vi "2100_Sequenced_Load Line w_Telegram Writes.vi"(0 "Semiconductor Module Context":T2, 1 "Published_Data_ID":string="HV_", 2 "Reg0_State":string="State00", 3 "HV_Load_Steps_uA":dbl[](array[numeric])=[0.0, 2.0, 4.0, 6.0, 8.0, 10.0, 12.0, 14.0, 16.0, 18.0, 20.0] format="%#_6p", 4 "USID":T1 max=15, 6 "Measurement:Aperture Time":dbl=2.5e-05 format="%#_13p", 8 "current level range":dbl=0.0001 format="%#_13p") -> ()   [LabVIEW 2013]
uses:
  <vilib>/NI_TestStand_SemiconductorModule/NI_TestStand_Semiconductor_Module.lvlibp/PinMap/General/SemiconductorModuleContext.ctl
  Controls/USID.ctl
  <instrlib>/niHSDIO/niHSDIO.llb/niHSDIO_ctl Generation Mode Values (Ring).ctl
  <instrlib>/niDCPower/nidcpower.llb/niDCPower Source Mode.ctl
  <instrlib>/niDCPower/nidcpower.llb/niDCPower Output Function.ctl
  <instrlib>/niDCPower/nidcpower.llb/niDCPower Sense.ctl
  <instrlib>/niDCPower/nidcpower.llb/niDCPower Wait For Event - Event.ctl
  <instrlib>/niHSDIO/niHSDIO.llb/niHSDIO_ctl Trigger SW - TrigName Values (Ring).ctl
  <instrlib>/niHSDIO/niHSDIO.llb/niHSDIO_ctl Trigger SW - TrigIdentifier Values (Ring).ctl
  <vilib>/NI_TestStand_SemiconductorModule/NI_TestStand_Semiconductor_Module.lvlibp/PinMap/HSDIO/PinsToNIHSDIOSessions.vi
  <vilib>/NI_TestStand_SemiconductorModule/NI_TestStand_Semiconductor_Module.lvlibp/PinMap/DC Power/PinsToNIDCPowerSessions.vi
  <vilib>/NI_TestStand_SemiconductorModule/NI_TestStand_Semiconductor_Module.lvlibp/PinMap/Deprecated/PublishDataDoubleMultiplePinsSingleInstrument.vi
  <vilib>/NI_TestStand_SemiconductorModule/NI_TestStand_Semiconductor_Module.lvlibp
panel:
  in  "Source:Transient Response":i32(ring)=1039 items=["Slow"=1041, "Normal"=1038, "Fast"=1039, "Custom"=1042]
  out "actual count":i32
  out "Avg_Meas_HV":dbl[](array[numeric])
  in  "Scratch Pad":string="Script test\nrepeat 10\nGenerate BRGu2rAd133\nend repeat\nend Script"
  in  "Num_Iterations_Per_Load_Step":i32=20
  in  "Script_Run":string="Script LoadLine\nRepeat Until ScriptTrigger0\nGenerate BRGu2rAd133\nend repeat\nend Script"
  in  "HSDIO_Pins":string[](array[string])=["CLK", "SDA"]
  out "HV Load Current":cluster{"X":dbl, "Y":dbl}[](graph)=[{"X"=0.0, "Y"=-1.7168055552671937e-06}, {"X"=2.4999999999999998e-05, "Y"=2.162222413914116e-07}, {"X"=4.9999999999999996e-05, "Y"=1.90283128600777e-07}, {"X"=7.5e-05, "Y"=1.7674967844914135e-07}, {"X"=9.999999999999999e-05, "Y"=1.7674967844914135e-07}, {"X"=0.000125, "Y"=-9.183319963206986e-07}, {"X"=0.00015, "Y"=1.993054287018673e-07}, {"X"=0.00017499999999999997, "Y"=1.891553410881407e-07}, {"X"=0.00019999999999999998, "Y"=1.7900525347441391e-07}, {"X"=0.000225, "Y"=-1.190128786866045e-06}, {"X"=0.00025, "Y"=2.2298896646722935e-07}, {"X"=0.00027499999999999996, "Y"=1.993054287018673e-07}, {"X"=0.0003, "Y"=1.812608284996865e-07}, {"X"=0.000325, "Y"=1.812608284996865e-07}, {"X"=0.00034999999999999994, "Y"=-9.093096962196083e-07}, {"X"=0.00037499999999999995, "Y"=1.891553410881407e-07}, {"X"=0.00039999999999999996, "Y"=1.8689976606286793e-07}, {"X"=0.000425, "Y"=1.880275535755044e-07}, {"X"=0.00045, "Y"=-1.5837266287761109e-06}, {"X"=0.00047499999999999994, "Y"=2.3426684159359224e-07}, {"X"=0.0005, "Y"=1.8013304098705022e-07}, {"X"=0.000525, "Y"=1.7900525347441391e-07}, {"X"=0.0005499999999999999, "Y"=1.8351640352495906e-07}, {"X"=0.000575, "Y"=-6.634520184648964e-07}, {"X"=0.0006, "Y"=2.1283887885350274e-07}, {"X"=0.0006249999999999999, "Y"=1.9141091611341327e-07}, {"X"=0.00065, "Y"=1.7449410342386876e-07}, {"X"=0.0006749999999999999, "Y"=-9.792325220030581e-07}, {"X"=0.0006999999999999999, "Y"=1.812608284996865e-07}, {"X"=0.000725, "Y"=1.7562189093650507e-07}, {"X"=0.0007499999999999999, "Y"=1.7787746596177763e-07}, {"X"=0.000775, "Y"=1.8013304098705022e-07}, {"X"=0.0007999999999999999, "Y"=6.763595465470189e-07}, {"X"=0.0008249999999999999, "Y"=2.094555163155939e-07}, {"X"=0.00085, "Y"=1.993054287018673e-07}, {"X"=0.0008749999999999999, "Y"=1.8689976606286793e-07}, {"X"=0.0009, "Y"=-9.453988966239696e-07}, {"X"=0.0009249999999999999, "Y"=1.9141091611341327e-07}, {"X"=0.0009499999999999999, "Y"=1.8013304098705022e-07}, {"X"=0.000975, "Y"=1.711107408859599e-07}, {"X"=0.001, "Y"=-3.0707116447182816e-07}, {"X"=0.0010249999999999999, "Y"=1.5419392819641557e-07}, {"X"=0.00105, "Y"=1.8238861601232278e-07}, {"X"=0.001075, "Y"=1.711107408859599e-07}, {"X"=0.0010999999999999998, "Y"=1.6772737834805105e-07}, {"X"=0.001125, "Y"=-9.386321715481518e-07}, {"X"=0.00115, "Y"=1.8351640352495906e-07}, {"X"=0.0011749999999999998, "Y"=1.8238861601232278e-07}, {"X"=0.0012, "Y"=1.8464419103759537e-07}, {"X"=0.001225, "Y"=-1.4810979651262086e-06}, {"X"=0.0012499999999999998, "Y"=-1.13875834761234e-05}, {"X"=0.0012749999999999999, "Y"=-1.2762356454027042e-05}, {"X"=0.0013, "Y"=-1.1686447166972018e-05}, {"X"=0.0013249999999999998, "Y"=-1.2103728546647446e-05}, {"X"=0.0013499999999999999, "Y"=-1.1891704494271823e-05}, {"X"=0.001375, "Y"=-1.2064255983705175e-05}, {"X"=0.0013999999999999998, "Y"=-1.2136434384513899e-05}, {"X"=0.0014249999999999998, "Y"=-1.1844337418741099e-05}, {"X"=0.00145, "Y"=-1.1872532106557007e-05}, {"X"=0.001475, "Y"=-1.2131923234463352e-05}, {"X"=0.0014999999999999998, "Y"=-1.2065383771217813e-05}, {"X"=0.0015249999999999999, "Y"=-1.181050379336201e-05}, {"X"=0.00155, "Y"=-1.1981927495282728e-05}, {"X"=0.0015749999999999998, "Y"=-1.2099217396596903e-05}, {"X"=0.0015999999999999999, "Y"=-1.2056361471116722e-05}, {"X"=0.001625, "Y"=-1.2046211383502995e-05}, {"X"=0.0016499999999999998, "Y"=-1.1473295327083758e-05}, {"X"=0.0016749999999999998, "Y"=-1.2156734559741353e-05}, {"X"=0.0017, "Y"=-1.2094706246546357e-05}, {"X"=0.0017249999999999998, "Y"=-1.2060872621167267e-05}, {"X"=0.0017499999999999998, "Y"=-1.2048466958528269e-05}, {"X"=0.0017749999999999999, "Y"=-1.165825247915611e-05}, {"X"=0.0018, "Y"=-1.2139817747051807e-05}, {"X"=0.0018249999999999998, "Y"=-1.2071022708780994e-05}, {"X"=0.0018499999999999999, "Y"=-1.1707875129712107e-05}, {"X"=0.001875, "Y"=-1.2161245709791896e-05}, {"X"=0.0018999999999999998, "Y"=-1.2092450671521083e-05}, {"X"=0.0019249999999999998, "Y"=-1.2056361471116722e-05}, {"X"=0.00195, "Y"=-1.205410589609145e-05}, {"X"=0.0019749999999999998, "Y"=-1.1493595502311211e-05}, {"X"=0.002, "Y"=-1.2143201109589716e-05}, {"X"=0.002025, "Y"=-1.2102600759134812e-05}, {"X"=0.0020499999999999997, "Y"=-1.2065383771217813e-05}, {"X"=0.002075, "Y"=-1.192328254462564e-05}, {"X"=0.0021, "Y"=-1.1752986630217559e-05}, {"X"=0.0021249999999999997, "Y"=-1.212741208441281e-05}, {"X"=0.00215, "Y"=-1.2063128196192539e-05}, {"X"=0.002175, "Y"=-1.2048466958528269e-05}, {"X"=0.0021999999999999997, "Y"=-1.2043955808477724e-05}, {"X"=0.002225, "Y"=-1.1619907703726478e-05}, {"X"=0.00225, "Y"=-1.219056818512044e-05}, {"X"=0.0022749999999999997, "Y"=-1.2086811733957902e-05}, {"X"=0.0023, "Y"=-1.2062000408679905e-05}, {"X"=0.002325, "Y"=-1.205410589609145e-05}, {"X"=0.0023499999999999997, "Y"=-1.1803737068286193e-05}, {"X"=0.002375, "Y"=-1.2008994395585998e-05}, {"X"=0.0024, "Y"=-1.2109367484210629e-05}, {"X"=0.0024249999999999996, "Y"=-1.2065383771217813e-05}, {"X"=0.00245, "Y"=-1.2043955808477724e-05}, {"X"=0.0024749999999999998, "Y"=-1.1533068065253484e-05}, {"X"=0.0024999999999999996, "Y"=-1.2196207122683623e-05}, {"X"=0.002525, "Y"=-1.2089067308983174e-05}, {"X"=0.0025499999999999997, "Y"=-1.2064255983705175e-05}, {"X"=0.0025749999999999996, "Y"=-1.2047339171015633e-05}, {"X"=0.0026, "Y"=-1.1910876881986638e-05}, {"X"=0.0026249999999999997, "Y"=-1.1693213892047838e-05}, {"X"=0.0026499999999999996, "Y"=-1.2147712259640262e-05}, {"X"=0.002675, "Y"=-1.2067639346243084e-05}, {"X"=0.0026999999999999997, "Y"=-1.2051850321066179e-05}, {"X"=0.0027249999999999996, "Y"=-1.184772078127901e-05}, {"X"=0.00275, "Y"=-1.1878171044120186e-05}, {"X"=0.0027749999999999997, "Y"=-1.2128539871925444e-05}, {"X"=0.0027999999999999995, "Y"=-1.206989492126836e-05}, {"X"=0.002825, "Y"=-1.2056361471116722e-05}, {"X"=0.0028499999999999997, "Y"=-1.1917643607062459e-05}, {"X"=0.002875, "Y"=-1.1721408579863744e-05}, {"X"=0.0029, "Y"=-1.2137562172026535e-05}, {"X"=0.0029249999999999996, "Y"=-1.2063128196192539e-05}, {"X"=0.00295, "Y"=-1.2047339171015633e-05}, {"X"=0.0029749999999999998, "Y"=-1.1780053530520832e-05}, {"X"=0.0029999999999999996, "Y"=-1.1910876881986638e-05}, {"X"=0.003025, "Y"=-1.2121773146849627e-05}, {"X"=0.0030499999999999998, "Y"=-1.2063128196192539e-05}, {"X"=0.0030749999999999996, "Y"=-1.2042828020965086e-05}, {"X"=0.0031, "Y"=-1.2037189083401907e-05}, {"X"=0.0031249999999999997, "Y"=-1.1581562928296841e-05}, {"X"=0.0031499999999999996, "Y"=-1.2186057035069897e-05}, {"X"=0.003175, "Y"=-1.2082300583907356e-05}, {"X"=0.0031999999999999997, "Y"=-1.2049594746040903e-05}, {"X"=0.0032249999999999996, "Y"=-1.2046211383502995e-05}, {"X"=0.00325, "Y"=-1.1610885403625385e-05}, {"X"=0.0032749999999999997, "Y"=-1.2252596498315437e-05}, {"X"=0.0032999999999999995, "Y"=-1.2089067308983174e-05}, {"X"=0.003325, "Y"=-1.2067639346243084e-05}, {"X"=0.0033499999999999997, "Y"=-1.1626674428802295e-05}, {"X"=0.0033749999999999995, "Y"=-1.2208612785322621e-05}, {"X"=0.0034, "Y"=-1.2101472971622174e-05}, {"X"=0.0034249999999999997, "Y"=-1.2078917221369447e-05}, {"X"=0.0034499999999999995, "Y"=-1.1853359718842188e-05}, {"X"=0.003475, "Y"=-1.2004483245535455e-05}, {"X"=0.0034999999999999996, "Y"=-1.213305102197599e-05}, {"X"=0.0035249999999999995, "Y"=-1.2089067308983174e-05}, {"X"=0.0035499999999999998, "Y"=-1.2080045008882085e-05}, {"X"=0.0035749999999999996, "Y"=-1.1715769642300562e-05}, {"X"=0.0036, "Y"=-1.2038316870914541e-05}, {"X"=0.0036249999999999998, "Y"=-1.2115006421773808e-05}, {"X"=0.0036499999999999996, "Y"=-1.2073278283806268e-05}, {"X"=0.003675, "Y"=-1.2049594746040903e-05}]
  out "current measurements":dbl[](array[numeric])=[-1.7168055552671937e-06, 2.162222413914116e-07, 1.90283128600777e-07, 1.7674967844914135e-07, 1.7674967844914135e-07, -9.183319963206986e-07, 1.993054287018673e-07, 1.891553410881407e-07, 1.7900525347441391e-07, -1.190128786866045e-06, 2.2298896646722935e-07, 1.993054287018673e-07, 1.812608284996865e-07, 1.812608284996865e-07, -9.093096962196083e-07, 1.891553410881407e-07, 1.8689976606286793e-07, 1.880275535755044e-07, -1.5837266287761109e-06, 2.3426684159359224e-07, 1.8013304098705022e-07, 1.7900525347441391e-07, 1.8351640352495906e-07, -6.634520184648964e-07, 2.1283887885350274e-07, 1.9141091611341327e-07, 1.7449410342386876e-07, -9.792325220030581e-07, 1.812608284996865e-07, 1.7562189093650507e-07, 1.7787746596177763e-07, 1.8013304098705022e-07, 6.763595465470189e-07, 2.094555163155939e-07, 1.993054287018673e-07, 1.8689976606286793e-07, -9.453988966239696e-07, 1.9141091611341327e-07, 1.8013304098705022e-07, 1.711107408859599e-07, -3.0707116447182816e-07, 1.5419392819641557e-07, 1.8238861601232278e-07, 1.711107408859599e-07, 1.6772737834805105e-07, -9.386321715481518e-07, 1.8351640352495906e-07, 1.8238861601232278e-07, 1.8464419103759537e-07, -1.4810979651262086e-06, -1.13875834761234e-05, -1.2762356454027042e-05, -1.1686447166972018e-05, -1.2103728546647446e-05, -1.1891704494271823e-05, -1.2064255983705175e-05, -1.2136434384513899e-05, -1.1844337418741099e-05, -1.1872532106557007e-05, -1.2131923234463352e-05, -1.2065383771217813e-05, -1.181050379336201e-05, -1.1981927495282728e-05, -1.2099217396596903e-05, -1.2056361471116722e-05, -1.2046211383502995e-05, -1.1473295327083758e-05, -1.2156734559741353e-05, -1.2094706246546357e-05, -1.2060872621167267e-05, -1.2048466958528269e-05, -1.165825247915611e-05, -1.2139817747051807e-05, -1.2071022708780994e-05, -1.1707875129712107e-05, -1.2161245709791896e-05, -1.2092450671521083e-05, -1.2056361471116722e-05, -1.205410589609145e-05, -1.1493595502311211e-05, -1.2143201109589716e-05, -1.2102600759134812e-05, -1.2065383771217813e-05, -1.192328254462564e-05, -1.1752986630217559e-05, -1.212741208441281e-05, -1.2063128196192539e-05, -1.2048466958528269e-05, -1.2043955808477724e-05, -1.1619907703726478e-05, -1.219056818512044e-05, -1.2086811733957902e-05, -1.2062000408679905e-05, -1.205410589609145e-05, -1.1803737068286193e-05, -1.2008994395585998e-05, -1.2109367484210629e-05, -1.2065383771217813e-05, -1.2043955808477724e-05, -1.1533068065253484e-05, -1.2196207122683623e-05, -1.2089067308983174e-05, -1.2064255983705175e-05, -1.2047339171015633e-05, -1.1910876881986638e-05, -1.1693213892047838e-05, -1.2147712259640262e-05, -1.2067639346243084e-05, -1.2051850321066179e-05, -1.184772078127901e-05, -1.1878171044120186e-05, -1.2128539871925444e-05, -1.206989492126836e-05, -1.2056361471116722e-05, -1.1917643607062459e-05, -1.1721408579863744e-05, -1.2137562172026535e-05, -1.2063128196192539e-05, -1.2047339171015633e-05, -1.1780053530520832e-05, -1.1910876881986638e-05, -1.2121773146849627e-05, -1.2063128196192539e-05, -1.2042828020965086e-05, -1.2037189083401907e-05, -1.1581562928296841e-05, -1.2186057035069897e-05, -1.2082300583907356e-05, -1.2049594746040903e-05, -1.2046211383502995e-05, -1.1610885403625385e-05, -1.2252596498315437e-05, -1.2089067308983174e-05, -1.2067639346243084e-05, -1.1626674428802295e-05, -1.2208612785322621e-05, -1.2101472971622174e-05, -1.2078917221369447e-05, -1.1853359718842188e-05, -1.2004483245535455e-05, -1.213305102197599e-05, -1.2089067308983174e-05, -1.2080045008882085e-05, -1.1715769642300562e-05, -1.2038316870914541e-05, -1.2115006421773808e-05, -1.2073278283806268e-05, -1.2049594746040903e-05, -1.159509637844848e-05] format="%#_6p"
  out "voltage measurements":dbl[](array[numeric])=[41.400019787154584, 41.491719884993515, 41.449526588441856, 41.407333291890204, 41.36626514991326, 41.397206900717805, 41.46246586605103, 41.421960301361445, 41.38032958209715, 41.350512985867304, 41.48159349382112, 41.4377124654074, 41.39383143699368, 41.35220071772937, 41.448401433867154, 41.45065174301657, 41.40902102375227, 41.365702572625906, 41.349387831292596, 41.47034194807401, 41.42814865152235, 41.384267623108634, 41.34151174926962, 41.47259225722343, 41.44052535184417, 41.39889463257987, 41.35276329501673, 41.397206900717805, 41.458527825039546, 41.417459683062596, 41.37189092278681, 41.33082278080987, 41.47990576195905, 41.43714988812004, 41.394394014281026, 41.35220071772937, 41.391581127844255, 41.45627751589013, 41.41127133290169, 41.369640613637394, 41.33194793538458, 41.47202967993607, 41.429273806097065, 41.38764308683277, 41.34657494485582, 41.47371741179815, 41.44727627929244, 41.40508298274078, 41.36457741805119, 41.350512985867304, 41.350512985867304, 41.17555144949977, 41.243060723982424, 41.27569020664904, 41.266126392763994, 41.25993804260308, 41.29931845271796, 41.317320925913336, 41.247561342281266, 41.273439897499614, 41.29650556628119, 41.30494422559152, 41.243060723982424, 41.27569020664904, 41.297068143568545, 41.31338288490185, 41.27906567037317, 41.238560105683575, 41.27456505207432, 41.29313010255706, 41.30944484389036, 41.25825031074102, 41.26556381547664, 41.29031721612028, 41.27794051579846, 41.243060723982424, 41.27625278393639, 41.29481783441912, 41.310007421177716, 41.289754638832925, 41.23124660094796, 41.26893927920077, 41.29144237069499, 41.30156876186739, 41.24249814669507, 41.257687733453665, 41.28412886595937, 41.298193298143254, 41.31338288490185, 41.26556381547664, 41.231809178235316, 41.26837670191342, 41.286941752396146, 41.30156876186739, 41.307194534740944, 41.24474845584449, 41.273439897499614, 41.297068143568545, 41.31113257575243, 41.28581659782144, 41.23912268297094, 41.27794051579846, 41.29594298899383, 41.30944484389036, 41.32069638963747, 41.25374969244218, 41.2610631971778, 41.288629484258216, 41.30494422559152, 41.31113257575243, 41.238560105683575, 41.26162577446515, 41.2875043296835, 41.3077571120283, 41.31450803947656, 41.24924907414333, 41.262188351752506, 41.289754638832925, 41.30606938016623, 41.310007421177716, 41.227308559936475, 41.25825031074102, 41.28581659782144, 41.29875587543061, 41.31394546218921, 41.27456505207432, 41.24362330126978, 41.27681536122375, 41.298193298143254, 41.311695153039786, 41.27850309308581, 41.257687733453665, 41.2875043296835, 41.305506802878874, 41.27794051579846, 41.25712515616631, 41.28581659782144, 41.304381648304165, 41.30888226660301, 41.24418587855713, 41.274002474786975, 41.298193298143254, 41.31394546218921, 41.310007421177716, 41.238560105683575, 41.26950185648813, 41.29144237069499, 41.30831968931565, 41.285254020534076]
  out "HV Voltage":cluster{"X":dbl, "Y":dbl}[](graph)=[{"X"=0.0, "Y"=41.400019787154584}, {"X"=2.4999999999999998e-05, "Y"=41.491719884993515}, {"X"=4.9999999999999996e-05, "Y"=41.449526588441856}, {"X"=7.5e-05, "Y"=41.407333291890204}, {"X"=9.999999999999999e-05, "Y"=41.36626514991326}, {"X"=0.000125, "Y"=41.397206900717805}, {"X"=0.00015, "Y"=41.46246586605103}, {"X"=0.00017499999999999997, "Y"=41.421960301361445}, {"X"=0.00019999999999999998, "Y"=41.38032958209715}, {"X"=0.000225, "Y"=41.350512985867304}, {"X"=0.00025, "Y"=41.48159349382112}, {"X"=0.00027499999999999996, "Y"=41.4377124654074}, {"X"=0.0003, "Y"=41.39383143699368}, {"X"=0.000325, "Y"=41.35220071772937}, {"X"=0.00034999999999999994, "Y"=41.448401433867154}, {"X"=0.00037499999999999995, "Y"=41.45065174301657}, {"X"=0.00039999999999999996, "Y"=41.40902102375227}, {"X"=0.000425, "Y"=41.365702572625906}, {"X"=0.00045, "Y"=41.349387831292596}, {"X"=0.00047499999999999994, "Y"=41.47034194807401}, {"X"=0.0005, "Y"=41.42814865152235}, {"X"=0.000525, "Y"=41.384267623108634}, {"X"=0.0005499999999999999, "Y"=41.34151174926962}, {"X"=0.000575, "Y"=41.47259225722343}, {"X"=0.0006, "Y"=41.44052535184417}, {"X"=0.0006249999999999999, "Y"=41.39889463257987}, {"X"=0.00065, "Y"=41.35276329501673}, {"X"=0.0006749999999999999, "Y"=41.397206900717805}, {"X"=0.0006999999999999999, "Y"=41.458527825039546}, {"X"=0.000725, "Y"=41.417459683062596}, {"X"=0.0007499999999999999, "Y"=41.37189092278681}, {"X"=0.000775, "Y"=41.33082278080987}, {"X"=0.0007999999999999999, "Y"=41.47990576195905}, {"X"=0.0008249999999999999, "Y"=41.43714988812004}, {"X"=0.00085, "Y"=41.394394014281026}, {"X"=0.0008749999999999999, "Y"=41.35220071772937}, {"X"=0.0009, "Y"=41.391581127844255}, {"X"=0.0009249999999999999, "Y"=41.45627751589013}, {"X"=0.0009499999999999999, "Y"=41.41127133290169}, {"X"=0.000975, "Y"=41.369640613637394}, {"X"=0.001, "Y"=41.33194793538458}, {"X"=0.0010249999999999999, "Y"=41.47202967993607}, {"X"=0.00105, "Y"=41.429273806097065}, {"X"=0.001075, "Y"=41.38764308683277}, {"X"=0.0010999999999999998, "Y"=41.34657494485582}, {"X"=0.001125, "Y"=41.47371741179815}, {"X"=0.00115, "Y"=41.44727627929244}, {"X"=0.0011749999999999998, "Y"=41.40508298274078}, {"X"=0.0012, "Y"=41.36457741805119}, {"X"=0.001225, "Y"=41.350512985867304}, {"X"=0.0012499999999999998, "Y"=41.350512985867304}, {"X"=0.0012749999999999999, "Y"=41.17555144949977}, {"X"=0.0013, "Y"=41.243060723982424}, {"X"=0.0013249999999999998, "Y"=41.27569020664904}, {"X"=0.0013499999999999999, "Y"=41.266126392763994}, {"X"=0.001375, "Y"=41.25993804260308}, {"X"=0.0013999999999999998, "Y"=41.29931845271796}, {"X"=0.0014249999999999998, "Y"=41.317320925913336}, {"X"=0.00145, "Y"=41.247561342281266}, {"X"=0.001475, "Y"=41.273439897499614}, {"X"=0.0014999999999999998, "Y"=41.29650556628119}, {"X"=0.0015249999999999999, "Y"=41.30494422559152}, {"X"=0.00155, "Y"=41.243060723982424}, {"X"=0.0015749999999999998, "Y"=41.27569020664904}, {"X"=0.0015999999999999999, "Y"=41.297068143568545}, {"X"=0.001625, "Y"=41.31338288490185}, {"X"=0.0016499999999999998, "Y"=41.27906567037317}, {"X"=0.0016749999999999998, "Y"=41.238560105683575}, {"X"=0.0017, "Y"=41.27456505207432}, {"X"=0.0017249999999999998, "Y"=41.29313010255706}, {"X"=0.0017499999999999998, "Y"=41.30944484389036}, {"X"=0.0017749999999999999, "Y"=41.25825031074102}, {"X"=0.0018, "Y"=41.26556381547664}, {"X"=0.0018249999999999998, "Y"=41.29031721612028}, {"X"=0.0018499999999999999, "Y"=41.27794051579846}, {"X"=0.001875, "Y"=41.243060723982424}, {"X"=0.0018999999999999998, "Y"=41.27625278393639}, {"X"=0.0019249999999999998, "Y"=41.29481783441912}, {"X"=0.00195, "Y"=41.310007421177716}, {"X"=0.0019749999999999998, "Y"=41.289754638832925}, {"X"=0.002, "Y"=41.23124660094796}, {"X"=0.002025, "Y"=41.26893927920077}, {"X"=0.0020499999999999997, "Y"=41.29144237069499}, {"X"=0.002075, "Y"=41.30156876186739}, {"X"=0.0021, "Y"=41.24249814669507}, {"X"=0.0021249999999999997, "Y"=41.257687733453665}, {"X"=0.00215, "Y"=41.28412886595937}, {"X"=0.002175, "Y"=41.298193298143254}, {"X"=0.0021999999999999997, "Y"=41.31338288490185}, {"X"=0.002225, "Y"=41.26556381547664}, {"X"=0.00225, "Y"=41.231809178235316}, {"X"=0.0022749999999999997, "Y"=41.26837670191342}, {"X"=0.0023, "Y"=41.286941752396146}, {"X"=0.002325, "Y"=41.30156876186739}, {"X"=0.0023499999999999997, "Y"=41.307194534740944}, {"X"=0.002375, "Y"=41.24474845584449}, {"X"=0.0024, "Y"=41.273439897499614}, {"X"=0.0024249999999999996, "Y"=41.297068143568545}, {"X"=0.00245, "Y"=41.31113257575243}, {"X"=0.0024749999999999998, "Y"=41.28581659782144}, {"X"=0.0024999999999999996, "Y"=41.23912268297094}, {"X"=0.002525, "Y"=41.27794051579846}, {"X"=0.0025499999999999997, "Y"=41.29594298899383}, {"X"=0.0025749999999999996, "Y"=41.30944484389036}, {"X"=0.0026, "Y"=41.32069638963747}, {"X"=0.0026249999999999997, "Y"=41.25374969244218}, {"X"=0.0026499999999999996, "Y"=41.2610631971778}, {"X"=0.002675, "Y"=41.288629484258216}, {"X"=0.0026999999999999997, "Y"=41.30494422559152}, {"X"=0.0027249999999999996, "Y"=41.31113257575243}, {"X"=0.00275, "Y"=41.238560105683575}, {"X"=0.0027749999999999997, "Y"=41.26162577446515}, {"X"=0.0027999999999999995, "Y"=41.2875043296835}, {"X"=0.002825, "Y"=41.3077571120283}, {"X"=0.0028499999999999997, "Y"=41.31450803947656}, {"X"=0.002875, "Y"=41.24924907414333}, {"X"=0.0029, "Y"=41.262188351752506}, {"X"=0.0029249999999999996, "Y"=41.289754638832925}, {"X"=0.00295, "Y"=41.30606938016623}, {"X"=0.0029749999999999998, "Y"=41.310007421177716}, {"X"=0.0029999999999999996, "Y"=41.227308559936475}, {"X"=0.003025, "Y"=41.25825031074102}, {"X"=0.0030499999999999998, "Y"=41.28581659782144}, {"X"=0.0030749999999999996, "Y"=41.29875587543061}, {"X"=0.0031, "Y"=41.31394546218921}, {"X"=0.0031249999999999997, "Y"=41.27456505207432}, {"X"=0.0031499999999999996, "Y"=41.24362330126978}, {"X"=0.003175, "Y"=41.27681536122375}, {"X"=0.0031999999999999997, "Y"=41.298193298143254}, {"X"=0.0032249999999999996, "Y"=41.311695153039786}, {"X"=0.00325, "Y"=41.27850309308581}, {"X"=0.0032749999999999997, "Y"=41.257687733453665}, {"X"=0.0032999999999999995, "Y"=41.2875043296835}, {"X"=0.003325, "Y"=41.305506802878874}, {"X"=0.0033499999999999997, "Y"=41.27794051579846}, {"X"=0.0033749999999999995, "Y"=41.25712515616631}, {"X"=0.0034, "Y"=41.28581659782144}, {"X"=0.0034249999999999997, "Y"=41.304381648304165}, {"X"=0.0034499999999999995, "Y"=41.30888226660301}, {"X"=0.003475, "Y"=41.24418587855713}, {"X"=0.0034999999999999996, "Y"=41.274002474786975}, {"X"=0.0035249999999999995, "Y"=41.298193298143254}, {"X"=0.0035499999999999998, "Y"=41.31394546218921}, {"X"=0.0035749999999999996, "Y"=41.310007421177716}, {"X"=0.0036, "Y"=41.238560105683575}, {"X"=0.0036249999999999998, "Y"=41.26950185648813}, {"X"=0.0036499999999999996, "Y"=41.29144237069499}, {"X"=0.003675, "Y"=41.30831968931565}]
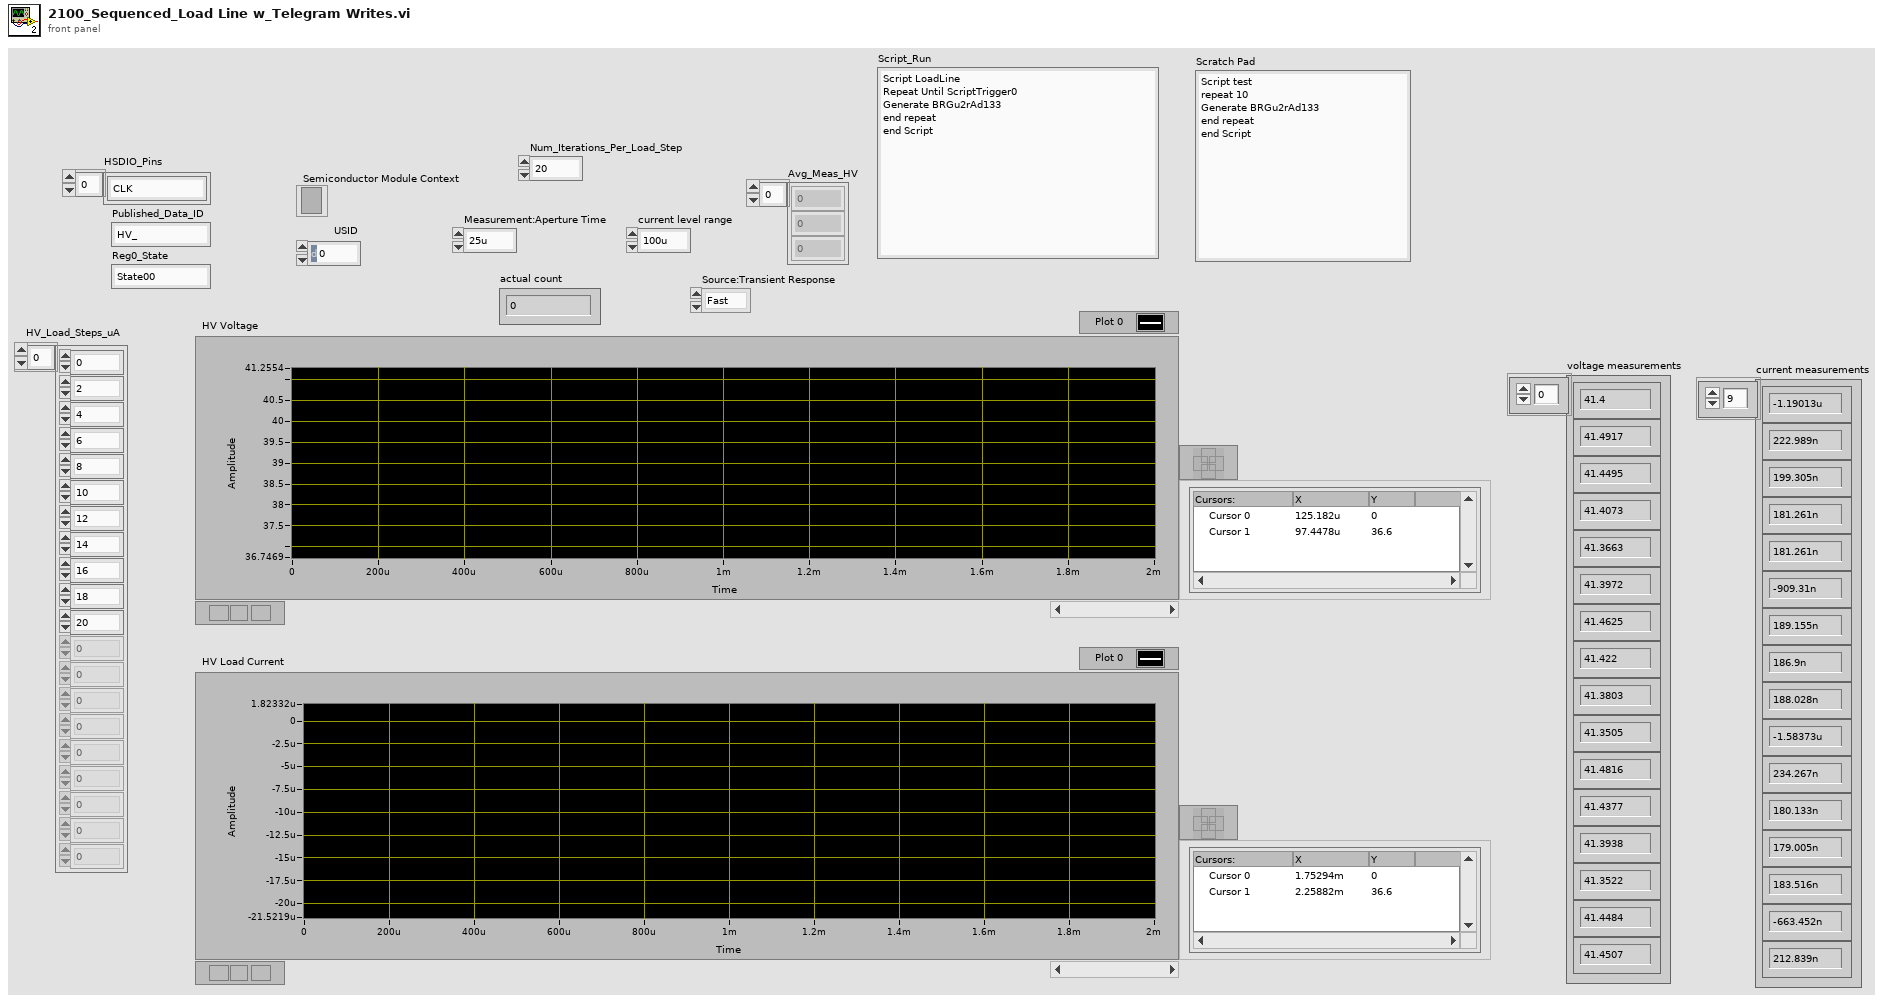
[diagram p1: front panel]
types:
  T1 = typedef "USID.ctl" = u8
  T2 = typedef "NI_TestStand_Semiconductor_Module.lvlibp/SemiconductorModuleContext.ctl" = refnum<k7>
  T3 = typedef "niHSDIO_ctl Generation Mode Values (Ring).ctl" = i32
  T4 = typedef "niHSDIO_ctl Trigger SW - TrigIdentifier Values (Ring).ctl" = string
  T5 = typedef "niHSDIO_ctl Trigger SW - TrigName Values (Ring).ctl" = i32
  T6 = typedef "niDCPower Source Mode.ctl" = i32
  T7 = typedef "niDCPower Wait For Event - Event.ctl" = i32
  T8 = typedef "niDCPower Sense.ctl" = i32
  T9 = typedef "niDCPower Output Function.ctl" = i32
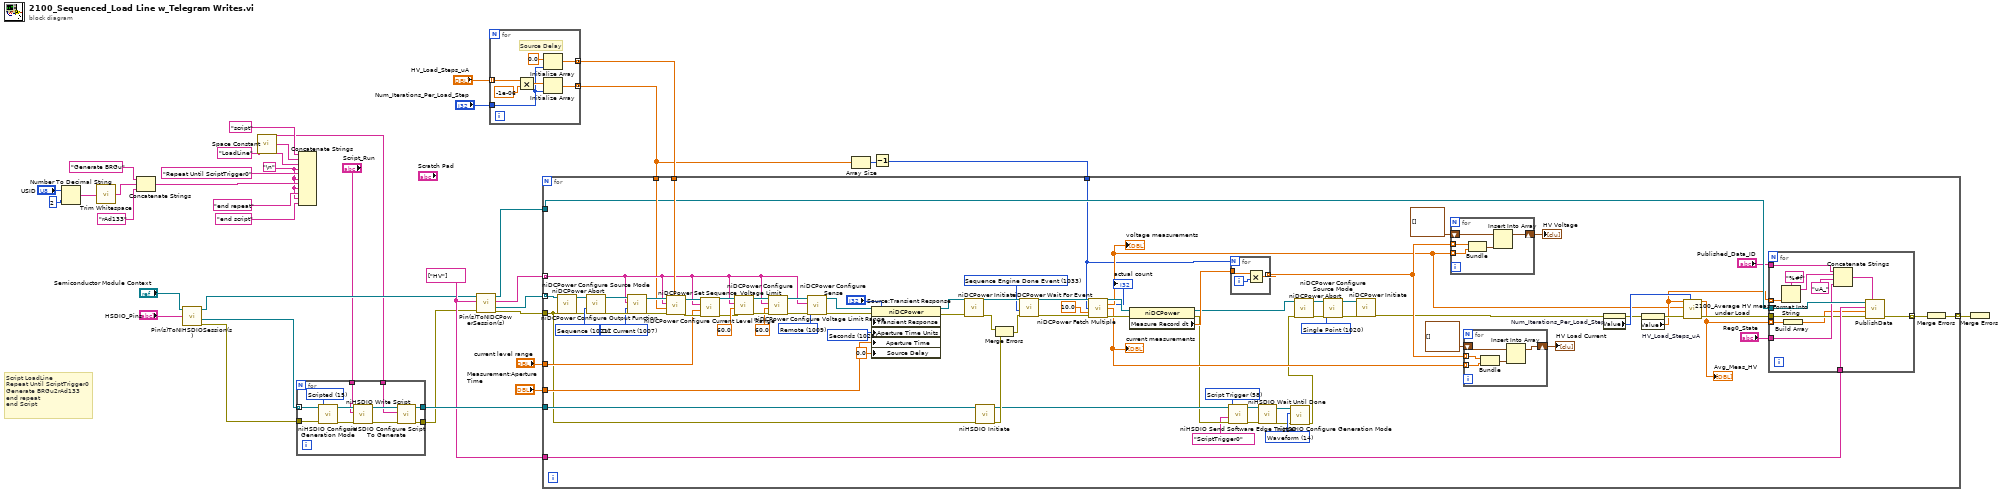
[diagram p0: block diagram]
diagram:
  w14 = "LoadLine" ("Script Name")
  w6 = "\n"
  w21 = string[] ["HV"] ("Pins")
  # "Script LoadLine\nRepeat Until ScriptTrigger0\nGenerate BRGu2rAd133\nend repeat\nend Script"
  n1 = Number To Decimal String(number="USID", width (-)=i16 2) -> (decimal integer string=w4:string)
  n2 = call <vilib>:"Trim Whitespace.vi"("string"=w4) -> ("trimmed string"=w3:string)  [unwired: 1 in]
  n3 = Concatenate Strings("Generate BRGu" ("Script Name"), w3, "rAd133" ("Script Name")) -> (w8:string)
  n4 = call-poly <vilib>:"Pin(s)ToNIHSDIOSession(s).vi"("Pins"="HSDIO_Pins", "Semiconductor Module Context"="Semiconductor Module Context") -> ("error out"=w26:errorcluster, "Generation Sessions"=w24:refnum<k15>[], "Semiconductor Module Context Out"=w17:T2)  [unwired: 4 in, 3 out]
  n5 = call <vilib>:"Space Constant.vi"() -> ("String"=w15:string)
  n6 = for {
    tunnel: w24 -> [w43] mode=indexing
    tunnel: w26 -> [w44]
    tunnel: [w40] -> w20
    tunnel: [w39] -> w23
    tunnel: w14 -> [w38]
    tunnel: "Script_Run" -> [w37]
    w45 = T3 15 items=["Waveform"=14, "Scripted"=15] ("generation mode (waveform)")
    n7 = call <instrlib>:"niHSDIO Configure Generation Mode.vi"("error in (no error)"=w44, "generation mode (waveform)"=w45, "instrument handle"=w43) -> ("error out"=w46:errorcluster, "instrument handle out"=w47:refnum<k15>)  [unwired: 7 in]
    n8 = call <instrlib>:"niHSDIO Write Script.vi"("error in (no error)"=w46, "script"=w37, "instrument handle"=w47) -> ("error out"=w42:errorcluster, "instrument handle out"=w41:refnum<k15>)  [unwired: 7 in]
    n9 = call <instrlib>:"niHSDIO Configure Script To Generate.vi"("error in (no error)"=w42, "script name"=w38, "instrument handle"=w41) -> ("error out"=w40:errorcluster, "instrument handle out"=w39:refnum<k15>)  [unwired: 7 in]
  }
  n10 = Concatenate Strings("script" ("string"), w15, w14, w6, "Repeat Until ScriptTrigger0" ("Script Name"), w6, w8, w6, "end repeat", w6, "end script") -> ()  [unwired: 1 out]
  n11 = call-poly <vilib>:"Pin(s)ToNIDCPowerSession(s).vi"("error in (no error)"=w20, "Pins"=w21, "Semiconductor Module Context"=w17) -> ("error out"=w36:errorcluster, "Instrument Sessions"=w35:refnum<k15>[], "Channel Lists"=w34:string[], "Semiconductor Module Context Out"=w22:T2)  [unwired: 4 in, 1 out]
  n12 = for {
    tunnel: "HV_Load_Steps_uA" -> [w51] mode=indexing
    tunnel: [w54] -> w28 mode=concatenating
    tunnel: "Num_Iterations_Per_Load_Step" -> [w48]
    tunnel: [w50] -> w32 mode=concatenating
    # "Source Delay"
    n13 = Multiply(x=w51, y=-1e-06) -> (x*y=w52:dbl)
    n14 = Initialize Array(0.0 ("element"), w48) -> (w50:dbl[])
    n15 = Initialize Array(w52, w48) -> (w54:dbl[])
  }
  n16 = Array Size(array=w28) -> (size(s)=w29:i32)
  n17 = Decrement(x=w29) -> (x-1=w27:i32)
  n18 = for {
    tunnel: w32 -> [w119]
    tunnel: w36 -> [w62]
    tunnel: w35 -> [w100] mode=indexing
    tunnel: w34 -> [w99] mode=indexing
    tunnel: w28 -> [w95]
    tunnel: "current level range" -> [w94]
    tunnel: "Measurement:Aperture Time" -> [w92]
    tunnel: w27 -> [w63]
    tunnel: w23 -> [w91]
    tunnel: w22 -> [w87]
    tunnel: w21 -> [w86]
    tunnel: [w78] -> w19 mode=indexing
    w57 = T5 58 items=["Start Trigger"=53, "Reference Trigger"=54, "Advance Trigger"=61, "Script Trigger"=58, "Stop Trigger"=82] ("trigger (start trigger)")
    w77 = T6 1020 items=["Single Point"=1020, "Sequence"=1021] ("source mode")
    w98 = T3 14 items=["Waveform"=14, "Scripted"=15] ("generation mode (waveform)")
    w103 = 1028 items=["Seconds"=1028, "Power Line Cycles"=1029] ("Measurement:Aperture Time Units")
    w104 = T7 1033 items=["Source Complete Event"=1030, "Measure Complete Event"=1031, "Sequence Iteration Complete Event"=1032, "Sequence Engine Done Event"=1033, "Pulse Complete Event"=1051, "Ready For Pulse Trigger Event"=1052] ("event")
    w107 = T8 1009 items=["Local"=1008, "Remote"=1009] ("sense")
    w134 = T9 1007 items=["DC Voltage"=1006, "DC Current"=1007, "Pulse Voltage"=1049, "Pulse Current"=1050] ("output function")
    w137 = T6 1021 items=["Single Point"=1020, "Sequence"=1021] ("source mode")
    n19 = call <instrlib>:"niDCPower Abort.vi"("error in (no error)"=w62, "instrument handle"=w100) -> ("error out"=w101:errorcluster, "instrument handle out"=w102:refnum<k15>)  [unwired: 8 in]
    n20 = call <instrlib>:"niDCPower Configure Source Mode.vi"("error in (no error)"=w101, "source mode"=w137, "instrument handle"=w102) -> ("error out"=w135:errorcluster, "instrument handle out"=w136:refnum<k15>)  [unwired: 7 out]
    n21 = call <instrlib>:"niDCPower Configure Output Function.vi"("error in (no error)"=w135, "output function"=w134, "channel name"=w99, "instrument handle"=w136) -> ("error out"=w127:errorcluster, "instrument handle out"=w126:refnum<k15>)  [unwired: 6 out]
    n22 = call <instrlib>:"niDCPower Set Sequence.vi"("source delays"=w119, "error in (no error)"=w127, "values"=w95, "channel name"=w99, "instrument handle"=w126) -> ("error out"=w118:errorcluster, "instrument handle out"=w115:refnum<k15>)  [unwired: 5 in]
    n23 = call <instrlib>:"niDCPower Configure Current Level Range.vi"("error in (no error)"=w118, "current level range"=w94, "channel name"=w99, "instrument handle"=w115) -> ("error out"=w117:errorcluster, "instrument handle out"=w116:refnum<k15>)  [unwired: 6 in]
    n24 = call <instrlib>:"niDCPower Configure Voltage Limit.vi"("error in (no error)"=w117, "voltage limit"=60.0, "channel name"=w99, "instrument handle"=w116) -> ("error out"=w124:errorcluster, "instrument handle out"=w125:refnum<k15>)  [unwired: 6 in]
    n25 = call <instrlib>:"niDCPower Configure Voltage Limit Range.vi"("error in (no error)"=w124, "voltage limit range"=60.0, "channel name"=w99, "instrument handle"=w125) -> ("error out"=w123:errorcluster, "instrument handle out"=w122:refnum<k15>)  [unwired: 6 in]
    n26 = call <instrlib>:"niDCPower Configure Sense.vi"("error in (no error)"=w123, "sense"=w107, "channel name"=w99, "instrument handle"=w122) -> ("error out"=w93:errorcluster, "instrument handle out"=w114:refnum<k15>)  [unwired: 6 in]
    n27 = property class="niDCPower"(reference=w114, error in=w93, "Transient Response"="Source:Transient Response", "Aperture Time Units"=w103, "Aperture Time"=w92, "Source Delay"=0.0 ("Source:Advanced:Source Delay")) -> (reference out=w113:refnum<k15>, error out=w68:errorcluster)
    n28 = call <instrlib>:"niDCPower Initiate.vi"("error in (no error)"=w68, "instrument handle"=w113) -> ("error out"=w67:errorcluster, "instrument handle out"=w106:refnum<k15>)  [unwired: 2 in, 6 out]
    n29 = call <instrlib>:"niHSDIO Initiate.vi"("error in (no error)"=w62, "instrument handle"=w91) -> ("error out"=w66:errorcluster, "instrument handle out"=w59:refnum<k15>)  [unwired: 8 in]
    n30 = Merge Errors(w67, w66) -> (w65:errorcluster)
    n31 = call <instrlib>:"niDCPower Wait For Event.vi"("error in (no error)"=w65, "event"=w104, "instrument handle"=w106) -> ("error out"=w70:errorcluster, "instrument handle out"=w105:refnum<k15>)  [unwired: 7 in]
    n32 = call <instrlib>:"niDCPower Fetch Multiple.vi"("instrument handle"=w105, "count (1)"=w63, "timeout (sec)"=10.0, "error in (no error)"=w70) -> ("actual count"=→"actual count":i32, "instrument handle out"=w132:refnum<k15>, "voltage measurements"=w81:dbl[], "current measurements"=w108:dbl[], "error out"=w133:errorcluster)  [unwired: 6 in, 1 out]
    "voltage measurements" <- w81
    "current measurements" <- w108
    n33 = property class="niDCPower"(reference=w132, error in=w133) -> (reference out=w76:refnum<k15>, error out=w58:errorcluster, "Measure Record dt"=w131:dbl)
    n34 = call <instrlib>:"niHSDIO Send Software Edge Trigger.vi"("error in (no error)"=w58, "trigger identifier (none)"=T4 "ScriptTrigger0", "trigger (start trigger)"=w57, "instrument handle"=w59) -> ("error out"=w60:errorcluster, "instrument handle out"=w61:refnum<k15>)  [unwired: 6 in]
    n35 = for {
      N: w63 -> [_]
      tunnel: w131 -> [w162]
      tunnel: [w161] -> w109 mode=indexing
      i -> [w163]
      n36 = Multiply(x=w162, y=w163) -> (x*y=w161:dbl)
    }
    n37 = call <instrlib>:"niHSDIO Wait Until Done.vi"("error in (no error)"=w60, "instrument handle"=w61) -> ("error out"=w97:errorcluster, "instrument handle out"=w96:refnum<k15>)  [unwired: 8 in]
    n38 = call <instrlib>:"niHSDIO Configure Generation Mode.vi"("error in (no error)"=w97, "generation mode (waveform)"=w98, "instrument handle"=w96) -> ("error out"=w69:errorcluster)  [unwired: 7 in, 1 out]
    n39 = call <instrlib>:"niDCPower Abort.vi"("error in (no error)"=w69, "instrument handle"=w76) -> ("error out"=w74:errorcluster, "instrument handle out"=w75:refnum<k15>)  [unwired: 8 in]
    n40 = call <instrlib>:"niDCPower Configure Source Mode.vi"("error in (no error)"=w74, "source mode"=w77, "instrument handle"=w75) -> ("error out"=w72:errorcluster, "instrument handle out"=w73:refnum<k15>)  [unwired: 7 out]
    n41 = call <instrlib>:"niDCPower Initiate.vi"("error in (no error)"=w72, "instrument handle"=w73) -> ("error out"=w71:errorcluster)  [unwired: 2 in, 7 out]
    n42 = for {
      shift-right: [w159] -> w129
      shift-left: cluster{"X":dbl, "Y":dbl}[] [] ("XY Graph") -> [w160]
      tunnel: w109 -> [w156] mode=indexing
      tunnel: w81 -> [w157] mode=indexing
      n43 = Bundle(w156, w157) -> (w158:cluster{dbl, dbl})  [unwired: 1 in]
      n44 = Insert Into Array(array=w160, new element=w158) -> (w159:cluster{"X":dbl, "Y":dbl}[])  [unwired: 1 in]
    }
    "HV Voltage" <- w129
    n45 = for {
      shift-right: [w154] -> w110
      shift-left: cluster{"X":dbl, "Y":dbl}[] [] ("XY Graph") -> [w155]
      tunnel: w109 -> [w151] mode=indexing
      tunnel: w108 -> [w152] mode=indexing
      n46 = Bundle(w151, w152) -> (w153:cluster{dbl, dbl})  [unwired: 1 in]
      n47 = Insert Into Array(array=w155, new element=w153) -> (w154:cluster{"X":dbl, "Y":dbl}[])  [unwired: 1 in]
    }
    "HV Load Current" <- w110
    n48 = property on="Num_Iterations_Per_Load_Step" class="DigNum (strict)"(error in=w71) -> (error out=w89:errorcluster, "Value"=w90:i32)  [unwired: 1 in, 1 out]
    n49 = property on="HV_Load_Steps_uA" class="Arr (strict)"(error in=w89) -> (error out=w88:errorcluster, "Value"=w82:dbl[])  [unwired: 1 in, 1 out]
    n50 = call "2100_Average HV meas under Load.vi"("Num_Iterations_Per_Load_Step"=w90, "Error In"=w88, "voltage measurements"=w81, "HV_Load_Steps_uA"=w82) -> ("Error Out"=w83:errorcluster, "Avg_Meas_HV"=w80:dbl[])  [unwired: 6 in]
    "Avg_Meas_HV" <- w80
    n51 = for {
      tunnel: "Published_Data_ID" -> [w144]
      tunnel: w82 -> [w148] mode=indexing
      tunnel: w87 -> [w147]
      tunnel: w86 -> [w145]
      tunnel: "Reg0_State" -> [w143]
      tunnel: w83 -> [w142]
      tunnel: [w141] -> w79 mode=indexing
      tunnel: w80 -> [w140] mode=indexing
      n52 = Format Into String(format string="%#f", w148) -> (resulting string=w138:string)  [unwired: 2 in, 1 out]
      n53 = Build Array(w140) -> (w139:dbl[])
      n54 = Concatenate Strings(w144, w138, "uA_" ("string"), w143) -> (w146:string)
      n55 = call-poly <vilib>:"PublishData.vi"("Measurement Id"=w146, "error in (no error)"=w142, "Data In"=w139, "Pins"=w145, "Semiconductor Module Context"=w147) -> ("error out"=w141:errorcluster)  [unwired: 5 in, 1 out]
    }
    n56 = Merge Errors(w79) -> (w78:errorcluster)
  }
  n57 = Merge Errors(w19) -> ()  [unwired: 1 out]
